vi "Get New Level.vi"(8 "error in (no error)":errorcluster, 11 "Cooler in":refnum<class "Cooler.lvclass">) -> (0 "error out":errorcluster, 2 "Level":dbl, 3 "Cooler out":refnum<class "Cooler.lvclass">)   [LabVIEW 2012, in "Cooler.lvlib" / "Cooler.lvclass"]
uses:
  Cooler.lvclass
  Cooler.lvclass/Cooler.ctl
  Cooler UI/Update Temperature Msg/Update Temperature Msg.lvclass/Update Temperature Msg.ctl
  <vilib>/ActorFramework/Message Enqueuer/Message Enqueuer.lvclass/Message Enqueuer.ctl
  <vilib>/ActorFramework/Message Enqueuer/Enqueue.vi
  Simulation/Simulation Data_Global.vi
  <vilib>/ActorFramework/Message Priority Queue/Priority Enqueue.vi
  Cooler UI/Update Temperature Msg/Update Temperature Msg.lvclass
  Simulation/Simulation.lvlib
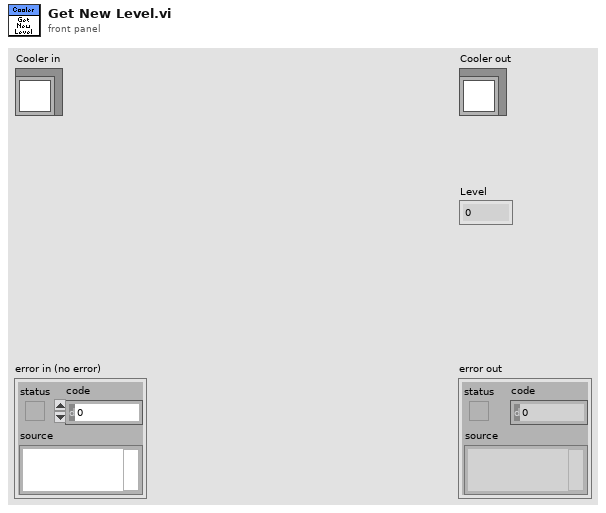
[diagram p1: front panel]
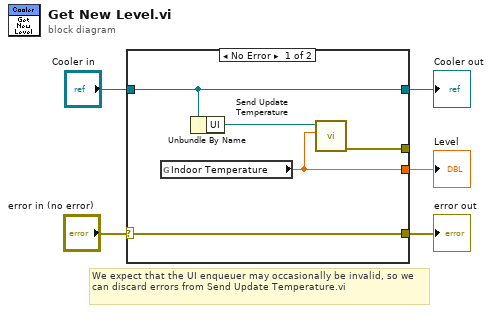
[diagram p0: block diagram]
diagram:
  # "We expect that the UI enqueuer may occasionally be invalid, so we can discard errors from Send Update Temperature.vi"
  n1 = case shown="No Error" "error in (no error)" {
    selector: "error in (no error)" -> [w8 w11]
    tunnel: "Cooler in" -> [w7 w12]
    tunnel: [w9 _] -> w4
    tunnel: [w8 w11] -> w2
    tunnel: [w7 w12] -> w1
    tunnel: [w6 _] -> _
    frame No Error {
      n2 = global read "Simulation Data_Global.vi" "Indoor Temperature"() -> (w9:dbl)
      n3 = Unbundle By Name(w7) -> ("UI"=w10:refnum<class "Message Enqueuer.lvclass">)
      n4 = call "Send Update Temperature.vi"("Level"=w9, "enqueuer"=w10) -> ("error out"=w6:errorcluster)  [unwired: 9 in]
    }
    frame Error {
    }
  }
  "error out" <- w2
  "Cooler out" <- w1
  "Level" <- w4
